vi "Acquire Data_SubVI.vi"(8 "error in (no error)":errorcluster, 11 "Configuration Settings":T1={"offset"=0.0, "Signal Type"=enum."Sine Wave", "Amplitude"=1.0, "Frequency"=10.0, "Phase"=0.0, "Noise Amplitude "=1.0} {"Noise Amplitude" format="%.2p"; "Phase" format="%.2p"; "Frequency" format="%0.2p"; "Amplitude" format="%0.2p"; "offset" format="%0.2p"}) -> (0 "error out":errorcluster, 3 "Data":dbl[](array[numeric]))   [LabVIEW 2020]
uses:
  <vilib>/measure/NI_MABase.lvlib
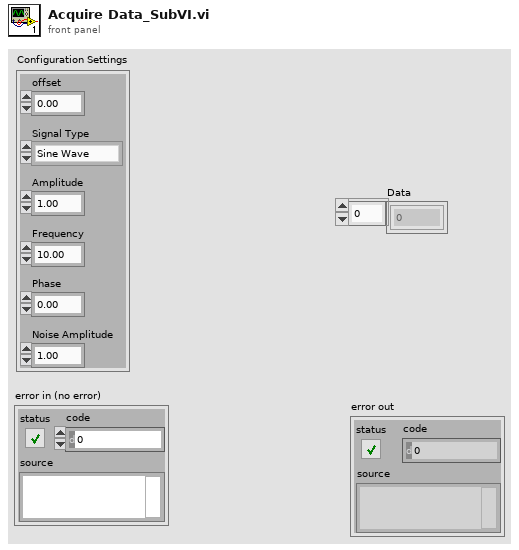
[diagram p1: front panel]
types:
  T1 = cluster{"offset":dbl, "Signal Type":enum16{"Sine Wave", "Triangle Wave", "Square Wave", "Sawtooth Wave"}, "Amplitude":dbl, "Frequency":dbl, "Phase":dbl, "Noise Amplitude ":dbl}
  T2 = enum16{"Sine Wave", "Triangle Wave", "Square Wave", "Sawtooth Wave"}
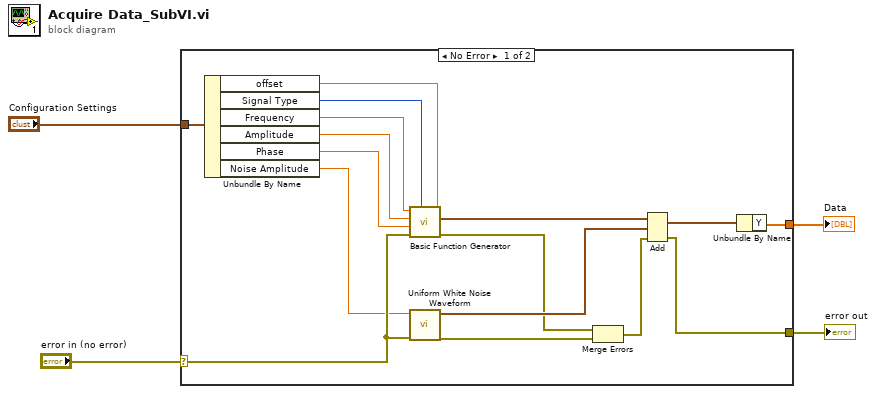
[diagram p0: block diagram]
diagram:
  n1 = case shown="No Error" "error in (no error)" {
    selector: "error in (no error)" -> [w13 w21]
    tunnel: [w17 _] -> w3
    tunnel: [w12 w21] -> w2
    tunnel: "Configuration Settings" -> [w5 _]
    frame No Error {
      n2 = Unbundle By Name(w5) -> ("offset"=w11:dbl, "Signal Type"=w10:T2, "Frequency"=w9:dbl, "Amplitude"=w8:dbl, "Phase"=w7:dbl, "Noise Amplitude"=w6:dbl)
      n3 = call <vilib>:"Basic Function Generator.vi"("offset"=w11, "signal type"=w10, "error in (no error)"=w13, "phase"=w7, "amplitude"=w8, "frequency"=w9) -> ("error out"=w15:errorcluster, "signal out"=w20:waveform(dbl))  [unwired: 3 in, 1 out]
      n4 = call <vilib>:"Uniform White Noise Waveform.vi"("error in (no error)"=w13, "amplitude"=w6) -> ("error out"=w14:errorcluster, "signal out"=w19:waveform(dbl))  [unwired: 8 in]
      n5 = Merge Errors(w15, w14) -> (w16:errorcluster)
      n6 = Add(1:w19, 2:w20, 4:w16) -> (0:w18:waveform(dbl), 3:w12:errorcluster)
      n7 = Unbundle By Name(w18) -> ("Y"=w17:dbl[])
    }
    frame Error {
    }
  }
  "error out" <- w2
  "Data" <- w3
